vi "PID Lead-Lag.vi"   [LabVIEW 2020, in "NI_PID_pid.lvlib"]
doc: "Implements a PID controller with a lead/lag function, which is generally used as a dynamic compensator in feedforward control schemes. This VI uses a positional algorithm and is an approximation of a true exponential lead/lag. Use the DBL instance of this VI to implement a single control loop. Use the DBL Array instance to implement parallel multi-loop control."
uses:
  <vilib>/addons/control/pid/NI_PID_pid.lvlib
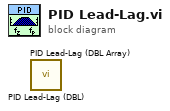
[diagram p0: block diagram]
diagram:
  n1 = call <vilib>:"PID Lead-Lag (DBL).vi"() -> ()  [unwired: 8 in, 2 out]
  n2 = call <vilib>:"PID Lead-Lag (DBL Array).vi"() -> ()  [unwired: 8 in, 2 out]
